vi "File dialog.vi"(8 "Multiselect":bool=TRUE, 9 "Prompt":string, 10 "Pattern":string, 11 "InitialDirectory":string) -> (1 "Cancelled":bool, 3 "FileNames":string[](array[string]))   [LabVIEW 2018]
uses:
  System.Windows.Forms
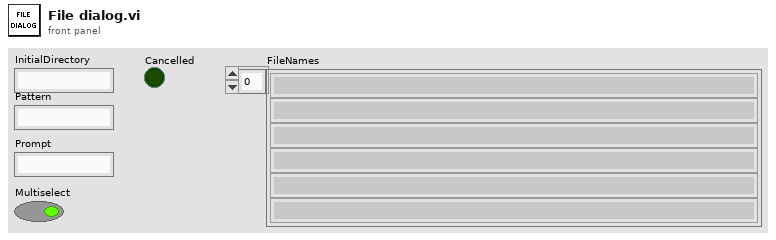
[diagram p1: front panel]
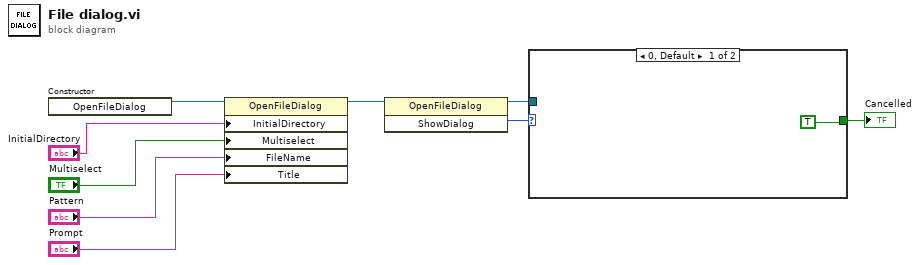
[diagram p0: block diagram]
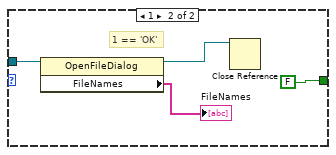
[diagram p2: hidden frame]
diagram:
  n1 = constructor class="OpenFileDialog"() -> (reference out=w9:refnum<k24>)  [unwired: 3 in, 2 out]
  n2 = property class="OpenFileDialog"(reference=w9, "InitialDirectory"="InitialDirectory", "Multiselect"="Multiselect", "FileName"="Pattern", "Title"="Prompt") -> (reference out=w6:refnum<k24>)  [unwired: 1 in, 1 out]
  n3 = invoke class="OpenFileDialog" method="ShowDialog"(reference=w6) -> (reference out=w8:refnum<k24>, "ShowDialog"=w7:i32)  [unwired: 2 in, 1 out]
  n4 = case shown="0, Default" w7 {
    tunnel: w8 -> [_ w14]
    tunnel: [TRUE FALSE] -> w1
    frame 0, Default {
    }
    frame 1 {
      # "1 == 'OK'"
      n5 = property class="OpenFileDialog"(reference=w14) -> (reference out=w13:refnum<k24>, "FileNames"=→"FileNames":string[])  [unwired: 1 in, 1 out]
      n6 = Close Reference(reference=w13) -> ()  [unwired: 1 in, 1 out]
    }
  }
  "Cancelled" <- w1
